vi "Differential_Drive_Kinematics_Speed_In.vi"(8 "Scale_Down_For_Turn":bool, 9 "Angular Speed(rad/s)":dbl, 10 "Linear_Speed(in/s)":dbl) -> (1 "Right_Motor_Velocity(rotations/s)":dbl, 2 "Left_Motor_Velocity(rotations/s)":dbl)   [LabVIEW 2019]
panel:
  in  "Gear_Reduction(output/input)":dbl=1.0
  in  "Wheel_Base_Radius(in)":dbl=11.87
  in  "Wheel_Radius(in)":dbl=3.0
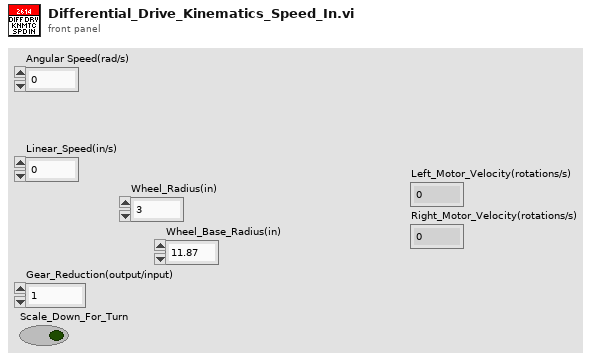
[diagram p1: front panel]
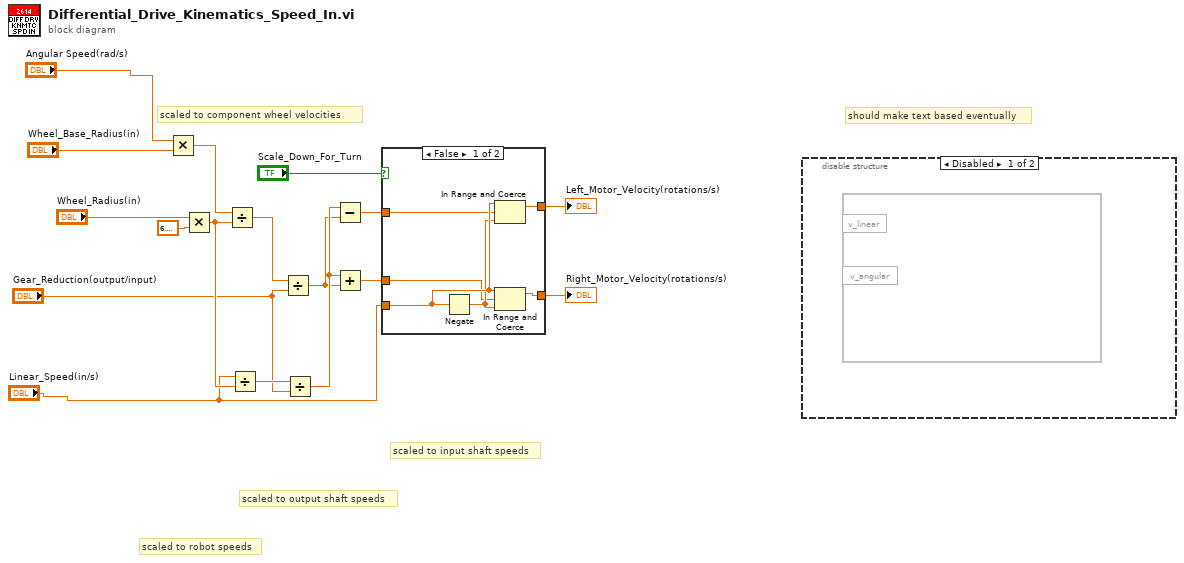
[diagram p0: block diagram]
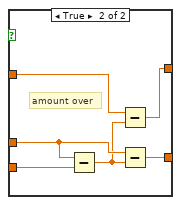
[diagram p3: hidden frame]
diagram:
  # "should make text based eventually"
  # "scaled to component wheel velocities"
  # "scaled to input shaft speeds"
  # "scaled to output shaft speeds"
  # "scaled to robot speeds"
  n1 = Multiply(x="Angular Speed(rad/s)", y="Wheel_Base_Radius(in)") -> (x*y=w13:dbl)
  n2 = Multiply(x="Wheel_Radius(in)", y=6.283185307179586) -> (x*y=w12:dbl)
  n3 = Divide(x=w13, y=w12) -> (x/y=w11:dbl)
  n4 = Divide(x="Linear_Speed(in/s)", y=w12) -> (x/y=w15:dbl)
  n5 = Divide(x=w11, y="Gear_Reduction(output/input)") -> (x/y=w8:dbl)
  n6 = Divide(x=w15, y="Gear_Reduction(output/input)") -> (x/y=w9:dbl)
  n7 = Subtract(x=w9, y=w8) -> (x-y=w6:dbl)
  n8 = Add(x=w9, y=w8) -> (x+y=w5:dbl)
  n9 = case shown="False" "Scale_Down_For_Turn" {
    tunnel: "Linear_Speed(in/s)" -> [w23 w29]
    tunnel: w6 -> [w21 w26]
    tunnel: w5 -> [w20 w27]
    tunnel: [w19 w28] -> w4
    tunnel: [w18 w24] -> w3
    frame False {
      n10 = Negate(x=w23) -> (-x=w22:dbl)
      n11 = In Range and Coerce(upper limit=w23, x=w21, lower limit=w22) -> (coerced(x)=w18:dbl)  [unwired: 1 out]
      n12 = In Range and Coerce(upper limit=w23, x=w20, lower limit=w22) -> (coerced(x)=w19:dbl)  [unwired: 1 out]
    }
    frame True {
      # "amount over"
      n13 = Subtract(x=w27, y=w29) -> (x-y=w25:dbl)
      n14 = Subtract(x=w26, y=w25) -> (x-y=w24:dbl)
      n15 = Subtract(x=w27, y=w25) -> (x-y=w28:dbl)
    }
  }
  "Right_Motor_Velocity(rotations/s)" <- w4
  "Left_Motor_Velocity(rotations/s)" <- w3
  n16 = disable-structure shown="Disabled" {
    frame Disabled {
      n17 = formula code=""() -> ()  [unwired: 2 in]
    }
    frame Enabled {
    }
  }
